vi "Shooter and Intake.vi"() -> ()   [LabVIEW 2011]
uses:
  Globals/Jaguar Commands.vi
  Globals/Robot Build.vi
  Globals/Shooter Speed Error.vi
  Globals/Shooter Gathering Velocity.vi
  Globals/Shooter Testing.vi
  Globals/Calculated Shooter Speed.vi
panel:
  in  "Uber Speed":dbl=12500.0
  in  "Fender Speed":dbl=5800.0
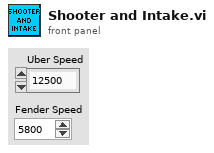
[diagram p1: front panel]
types:
  T1 = typedef "WPI_JoystickDevRef.ctl" = cluster{"Device":T2}
  T2 = typedef "WPI_JoystickDeviceEnum.ctl" = enum16{"USB 1", "USB 2", "USB 3", "USB 4", "Kinect 1", "Kinect 2"}
  T3 = typedef "WPI_JoystickButtonState.ctl" = cluster{"Button 1":bool, "Button 2":bool, "Button 3":bool, "Button 4":bool, "Button 5":bool, "Button 6":bool, "Button 7":bool, "Button 8":bool, "Button 9":bool, "Button 10":bool, "Button 11":bool, "Button 12":bool}
  T4 = cluster{"axis 1 (x)":dbl, "axis 2 (y)":dbl, "axis 3 (throttle)":dbl, "axis 4":dbl, "axis 5":dbl, "axis 6":dbl}
  T5 = typedef "Robot Build.ctl" = enum16{"Practice Bot", "Competition Bot"}
  T6 = typedef "WPI_MotorControlDeviceRef.ctl" = cluster{"DeviceStatus":errorcluster, "Type":enum16{"PWM", "CAN"}, "PWM":cluster{"Digital Module":T7, "PWM Channel":T8, "DeadBand":T9}, "CAN":cluster{"Device Number":u8, "Control Mode":T10, "Semaphore":T11, "Max Vout":dbl}, "Invert":bool, "TransformRef":T12, "InvTransformRef":T12}
  T7 = typedef "FPGA_TypedefDigitalModule.ctl" = enum16{"Digital Module 1", "Digital Module 2"}
  T8 = typedef "FPGA_DIOPWMChannel.ctl" = enum8{"PWM 1", "PWM 2", "PWM 3", "PWM 4", "PWM 5", "PWM 6", "PWM 7", "PWM 8", "PWM 9", "PWM 10", "Invalid"}
  T9 = typedef "WPI_PWMDeadband.ctl" = cluster{"Name":string, "maxPositivePwm":i32, "minPositivePwm":i32, "centerPwm":i32, "maxNegativePwm":i32, "minNegativePwm":i32, "angularRange":u16}
  T10 = typedef "WPI_CANJaguar_ControlMode.ctl" = enum8{"Percent VBus", "Current", "Speed", "Position", "Voltage"}
  T11 = typedef "Semaphore RefNum" = refnum<k1>
  T12 = typedef "WPI_PWMTransform_ConPane.ctl" = refnum<vi>
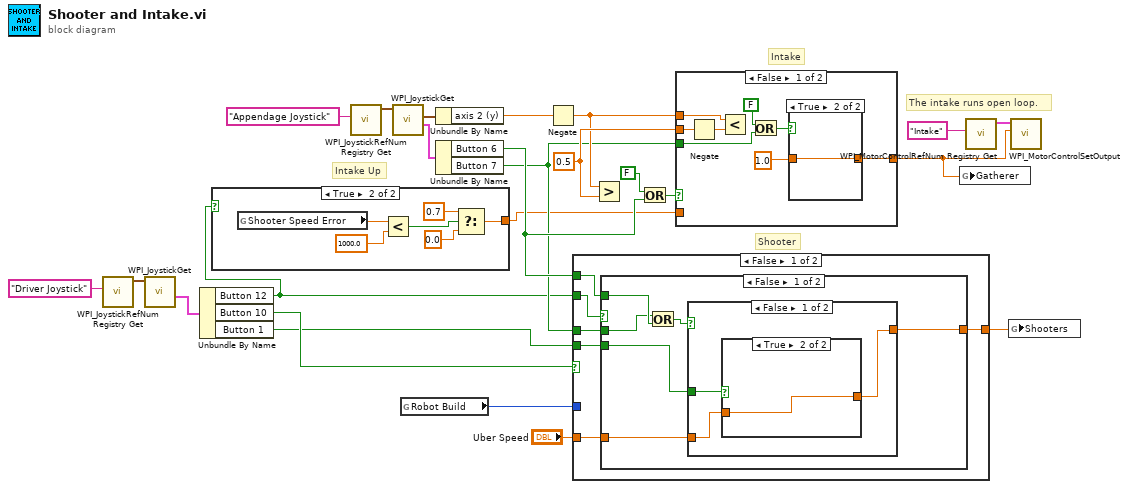
[diagram p0: block diagram]
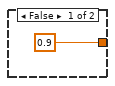
[diagram p2: hidden frame]
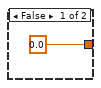
[diagram p3: hidden frame]
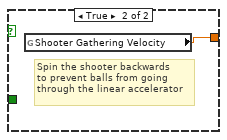
[diagram p4: hidden frame]
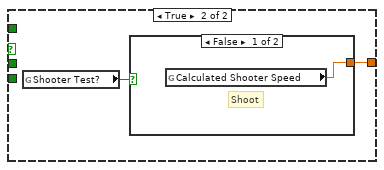
[diagram p5: hidden frame]
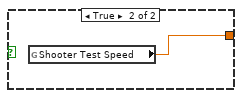
[diagram p6: hidden frame]
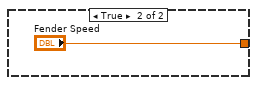
[diagram p7: hidden frame]
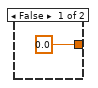
[diagram p8: hidden frame]
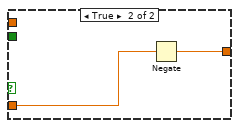
[diagram p9: hidden frame]
diagram:
  w17 = 0.5 ("y")
  # "Intake Up"
  # "Shooter"
  # "Intake"
  # "The intake runs open loop."
  n1 = call <vilib>:"WPI_JoystickRefNum Registry Get.vi"("refnum name"="Driver Joystick") -> ("JoystickDevRef"=w13:T1)  [unwired: 9 in, 1 out]
  n2 = call <vilib>:"WPI_JoystickGet.vi"("JoystickDevRef"=w13) -> ("Buttons"=w12:T3)  [unwired: 4 in, 2 out]
  n3 = Unbundle By Name(w12) -> ("Button 12"=w1:bool, "Button 10"=w9:bool, "Button 1"=w5:bool)
  n4 = case shown="True" w1 {
    tunnel: [0.9 ("upper limit") w31] -> w2
    frame False {
    }
    frame True {
      n5 = global read "Shooter Speed Error.vi" "Shooter Speed Error"() -> (w30:dbl)
      n6 = Less?(x=w30, y=1000.0) -> (x < y?=w26:bool)
      n7 = Select(t=0.7, s=w26, f=0.0) -> (s? t:f=w31:dbl)
    }
  }
  n8 = call <vilib>:"WPI_JoystickRefNum Registry Get.vi"("refnum name"="Appendage Joystick") -> ("JoystickDevRef"=w21:T1)  [unwired: 9 in, 1 out]
  n9 = call <vilib>:"WPI_JoystickGet.vi"("JoystickDevRef"=w21) -> ("Buttons"=w24:T3, "Axes"=w22:T4)  [unwired: 4 in, 1 out]
  n10 = global read "Robot Build.vi" "Robot Build"() -> (w7:T5)
  n11 = Unbundle By Name(w22) -> ("axis 2 (y)"=w23:dbl)
  n12 = Unbundle By Name(w24) -> ("Button 6"=w8:bool, "Button 7"=w3:bool)
  n13 = Negate(x=w23) -> (-x=w16:dbl)
  n14 = case shown="False" w9 {
    tunnel: w1 -> [w37 _]
    tunnel: [w36 "Fender Speed"] -> w11
    tunnel: w8 -> [w35 _]
    tunnel: w7 -> [_ _]
    tunnel: "Uber Speed" -> [w34 _]
    tunnel: w5 -> [w33 _]
    tunnel: w3 -> [w32 _]
    frame False {
      n15 = case shown="False" w37 {
        tunnel: [w43 w51] -> w36
        tunnel: w35 -> [w42 _]
        tunnel: w34 -> [w41 _]
        tunnel: w33 -> [w40 _]
        tunnel: w32 -> [w38 _]
        frame False {
          n16 = Or(x=w38, y=w42) -> (x .or. y?=w39:bool)
          n17 = case shown="False" w39 {
            tunnel: [w46 w49] -> w43
            tunnel: w41 -> [w45 _]
            tunnel: w40 -> [w44 _]
            frame False {
              n18 = case shown="True" w44 {
                tunnel: [0.0 w48] -> w46
                tunnel: w45 -> [_ w48]
                frame False {
                }
                frame True {
                }
              }
            }
            frame True {
              # "Spin the shooter backwards\nto prevent balls from going\nthrough the linear accelerator"
              n19 = global read "Shooter Gathering Velocity.vi" "Shooter Gathering Velocity"() -> (w49:dbl)
            }
          }
        }
        frame True {
          n20 = global read "Shooter Testing.vi" "Shooter Test?"() -> (w50:bool)
          n21 = case shown="False" w50 {
            tunnel: [w52 w53] -> w51
            frame False {
              # "Shoot"
              n22 = global read "Calculated Shooter Speed.vi" "Calculated Shooter Speed"() -> (w52:dbl)
            }
            frame True {
              n23 = global read "Shooter Testing.vi" "Shooter Test Speed"() -> (w53:dbl)
            }
          }
        }
      }
    }
    frame True {
    }
  }
  n24 = Greater?(x=w16, y=w17) -> ()  [unwired: 1 out]
  n25 = Or(x=FALSE, y=w8) -> (x .or. y?=w15:bool)
  n26 = case shown="False" w15 {
    tunnel: [w59 w66] -> w10
    tunnel: w17 -> [w62 _]
    tunnel: w16 -> [w60 _]
    tunnel: w3 -> [w58 _]
    tunnel: w2 -> [_ w65]
    frame False {
      n27 = Negate(x=w62) -> (-x=w61:dbl)
      n28 = Less?(x=w60, y=w61) -> ()  [unwired: 1 out]
      n29 = Or(x=FALSE, y=w58) -> (x .or. y?=w57:bool)
      n30 = case shown="True" w57 {
        tunnel: 1.0 -> [_ w64]
        tunnel: [0.0 w64] -> w59
        frame False {
        }
        frame True {
        }
      }
    }
    frame True {
      n31 = Negate(x=w65) -> (-x=w66:dbl)
    }
  }
  n32 = global write "Jaguar Commands.vi" "Gatherer"(w10) -> ()
  n33 = call <vilib>:"WPI_MotorControlRefNum Registry Get.vi"("refnum name"="Intake") -> ("MotorControlDevRef"=w18:T6)  [unwired: 9 in, 1 out]
  n34 = global write "Jaguar Commands.vi" "Shooters"(w11) -> ()
  n35 = call <vilib>:"WPI_MotorControlSetOutput.vi"("Output"=w10, "MotorControlDevRef"=w18) -> ()  [unwired: 8 in, 2 out]
